vi "miopen.vi"(2 "错误输入（无错误）":errorcluster, 3 "name":string, 4 "port":u16=1234, 5 "ip":string="127.0.0.1") -> (0 "错误输出":errorcluster, 1 "VISA资源名称输出":refnum<visa-resource-name>)   [LabVIEW 2017]
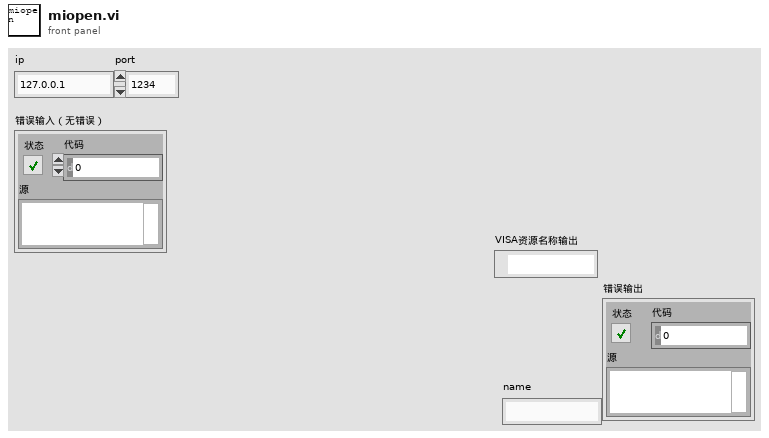
[diagram p1: front panel]
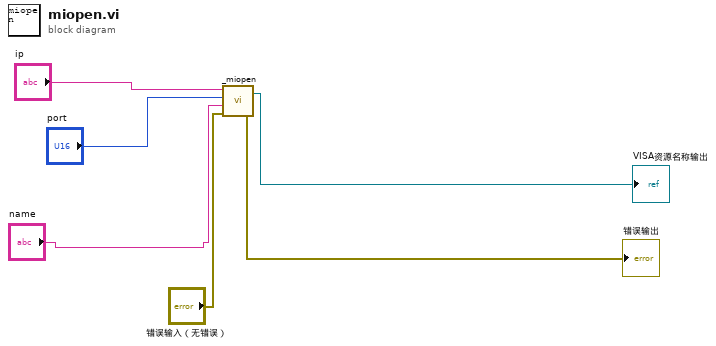
[diagram p0: block diagram]
diagram:
  n1 = call "_miopen.vi"("错误输入（无错误）"="错误输入（无错误）", "name"="name", "port"="port", "ip"="ip") -> ("错误输出"=→"错误输出":errorcluster, "VISA引用句柄输出"=→"VISA资源名称输出":refnum<visa-resource-name>)
